vi "RunAllTests.vi"() -> ()   [LabVIEW 2019]
panel:
  out "All Tests Finished":bool
  out "Geometry Util":bool
  # "FORMAL PathPlannerLib LabVIEW TEST PROCEDURE"
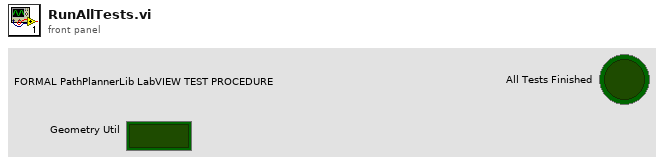
[diagram p1: front panel]
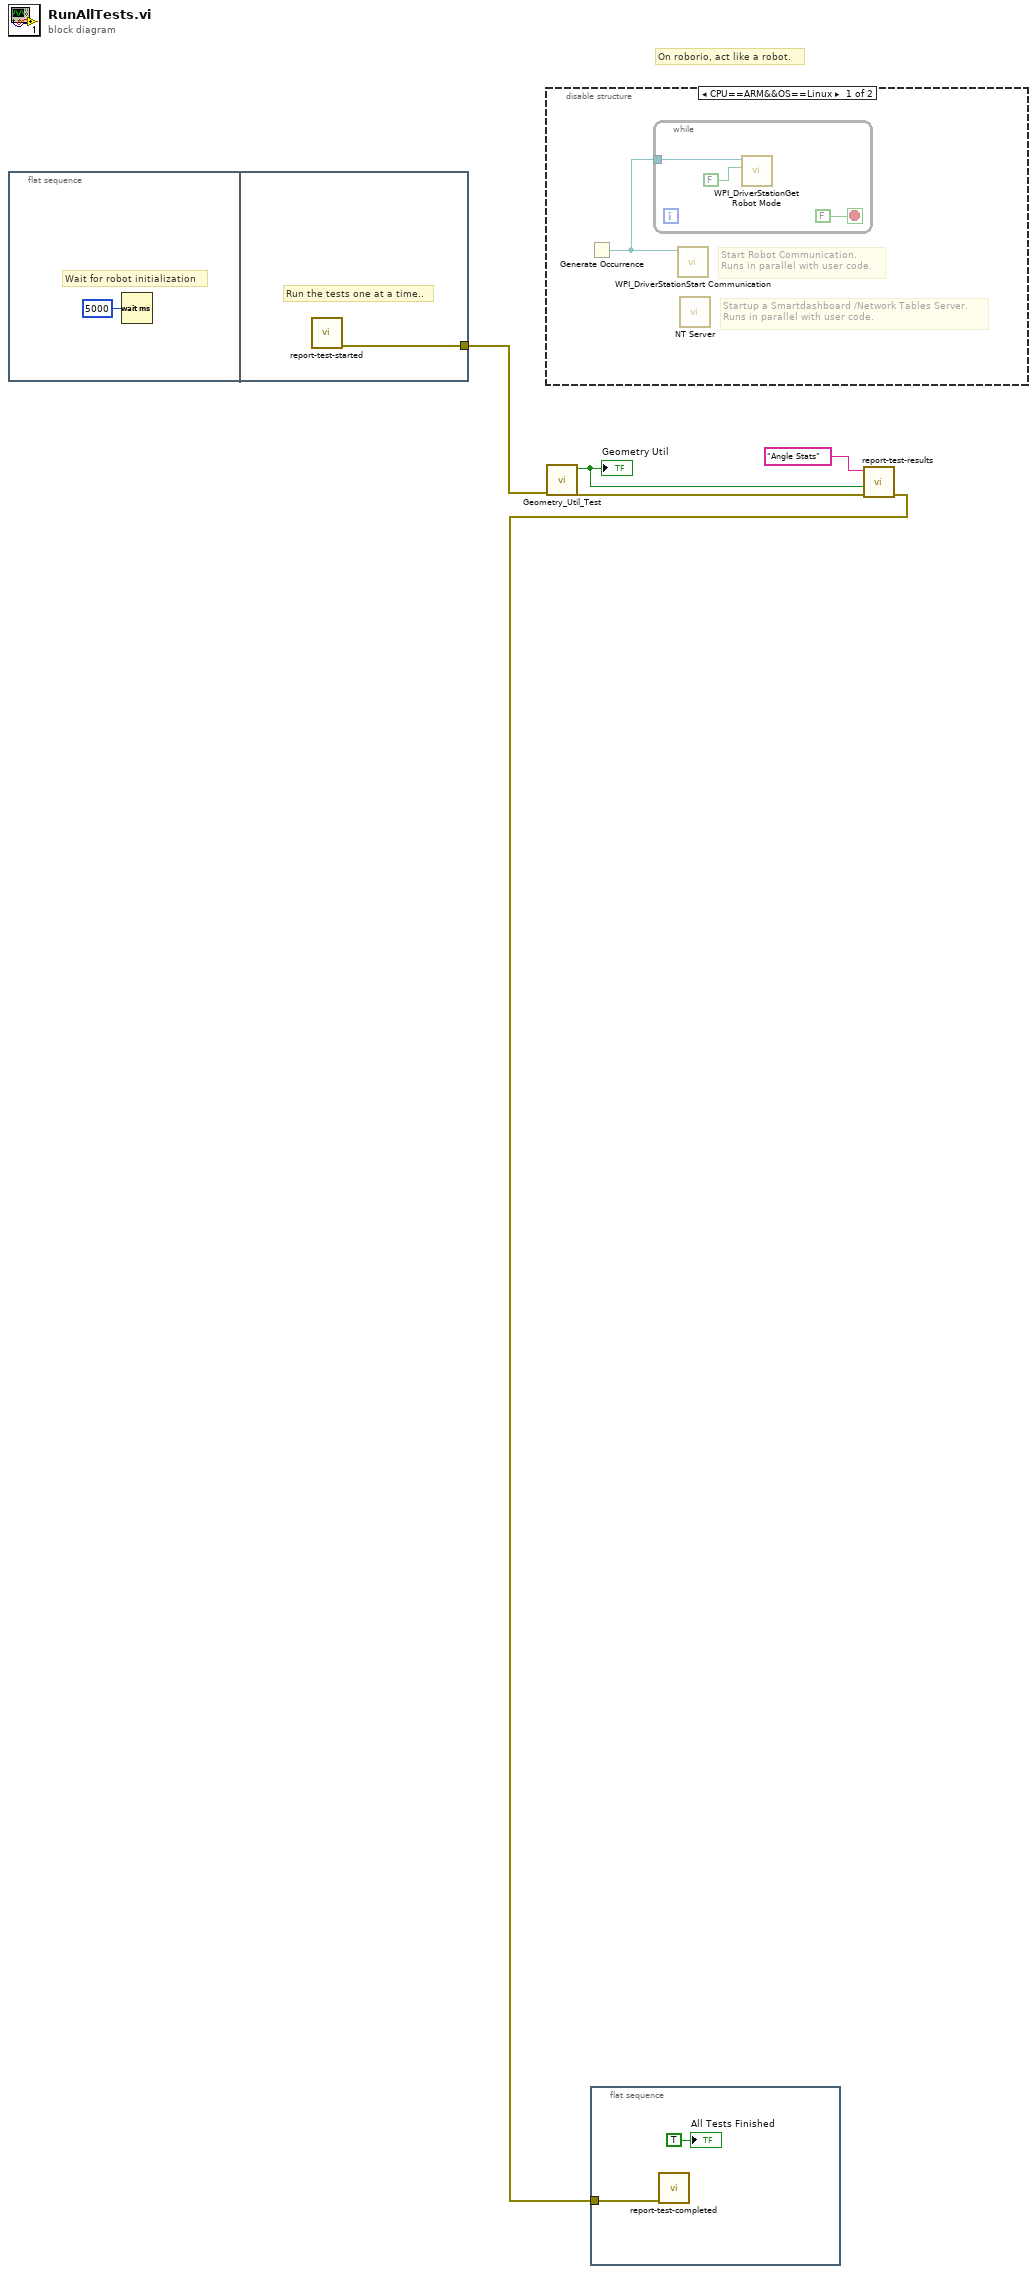
[diagram p0: block diagram]
diagram:
  # "On roborio, act like a robot."
  n1 = flat-sequence {
    tunnel: [w7] -> w2
    frame #0 {
      # "Wait for robot initialization"
      n2 = Wait (ms)(milliseconds to wait=u32 5000) -> ()  [unwired: 1 out]
    }
    frame #1 {
      # "Run the tests one at a time.."
      n3 = call "report-test-started.vi"() -> ("error out"=w7:errorcluster)  [unwired: 11 in]
    }
  }
  n4 = disable-structure shown="CPU==ARM&&OS==Linux" {
    frame condition #0 {
      # "Startup a Smartdashboard /Network Tables Server.\nRuns in parallel with user code."
      # "Start Robot Communication.\nRuns in parallel with user code."
      n5 = Generate Occurrence() -> (w8:refnum<k4>)
      n6 = while {
        tunnel: w8 -> [w11]
        stop <- FALSE stop-if-true
        n7 = call <vilib>:"WPI_DriverStationGet Robot Mode.vi"("Finish"=FALSE, "DS Occurrence"=w11) -> ()  [unwired: 10 out]
      }
      n8 = call <vilib>:"WPI_DriverStationStart Communication.vi"("occurrence"=w8) -> ()  [unwired: 2 in, 9 out]
      n9 = call <vilib>:"NT Server.vi"() -> ()  [unwired: 11 in, 1 out]
    }
    frame condition #1 (active) {
    }
  }
  n10 = call "Geometry_Util_Test.vi"("error in (no error)"=w2) -> ("error out"=w3:errorcluster, "All Passed"=w5:bool)  [unwired: 9 in]
  "Geometry Util" <- w5
  n11 = flat-sequence {
    tunnel: w1 -> [w12]
    frame #0 {
      n12 = call "report-test-completed.vi"("error in (no error)"=w12) -> ()  [unwired: 10 in, 1 out]
      "All Tests Finished" <- TRUE ("All Tests Finished")
    }
  }
  n13 = call "report-test-results.vi"("error in (no error)"=w3, "TestPassed"=w5, "Test Name"="Angle Stats") -> ("error out"=w1:errorcluster)  [unwired: 8 in]
